vi "FT10_Fornax Switch Status Command.vi"(7 "Generator":T5="{\"Partition\":\"", 8 "Switch State":T1, 9 "Energy Channel ID":T2, 10 "Switch ID":T3, 11 "Source ID":T4) -> (3 "JSON Command":string)   [LabVIEW 2015]
uses:
  Controls/Control_Fornax Generator.ctl
  Controls/Control_Fornax Source ID.ctl
  Controls/Control_Fornax Switch ID.ctl
  Controls/Control_Fornax Energy Channel ID.ctl
  Controls/Control_Fornax Switch State.ctl
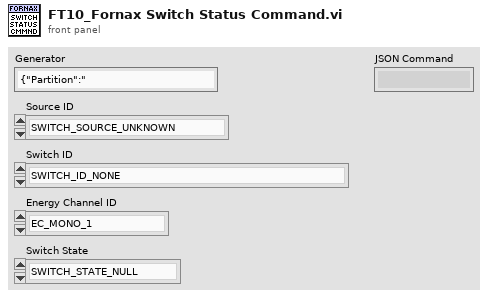
[diagram p1: front panel]
types:
  T1 = typedef "Control_Fornax Switch State.ctl" = enum16{"SWITCH_STATE_NULL  ", "SWITCH_STATE_PRESSED  ", "SWITCH_STATE_RELEASED  ", "NUM_SWITCH_STATES  "}
  T2 = typedef "Control_Fornax Energy Channel ID.ctl" = enum16{"EC_MONO_1  ", "EC_BIPOLAR  ", "EC_MONO_2  ", "EC_ADVANCED  ", "EC_ADVANCED_ECUT  ", "EC_ADVANCED_DCUT  ", "EC_SHARED_COAG  ", "EC_INTERNAL_BIP_CAL  "}
  T3 = typedef "Control_Fornax Switch ID.ctl" = enum16{"SWITCH_ID_NONE  ", "SWITCH_ID_CUT  ", "SWITCH_ID_VMODE  ", "SWITCH_ID_COAG  ", "SWITCH_ID_LIGASURE  ", "SWITCH_ID_BIPOLAR  ", "SWITCH_ID_STAPLER_CLOSE  ", "SWITCH_ID_STAPLER_OPEN  ", "SWITCH_ID_CARDIOBLATE_BIPOLAR  ", "SWITCH_ID_CARDIOBLATE_BIPOLAR_TOUCHSCREEN  ", "SWITCH_ID_CARDIOBLATE_MONOPOLAR  ", "SWITCH_ID_CARDIOBLATE_MONOPOLAR_TOUCHSCREEN  ", "SWITCH_ID_ULTRASONIC_BTN1  ", "SWITCH_ID_ULTRASONIC_BTN2  ", "SWITCH_ID_MAX  "}
  T4 = typedef "Control_Fornax Source ID.ctl" = enum16{"SWITCH_SOURCE_UNKNOWN  ", "SWITCH_SOURCE_HANDSWITCH  ", "SWITCH_SOURCE_FOOTSWITCH  ", "SWITCH_SOURCE_AUTO_BIPOLAR  ", "SWITCH_SOURCE_CARDIOBLATE  ", "SWITCH_SOURCE_SCREEN  ", "NUM_SWITCH_SOURCES  "}
  T5 = typedef "Control_Fornax Generator.ctl" = string
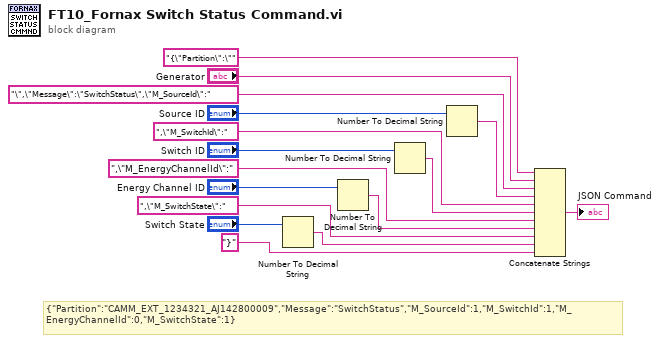
[diagram p0: block diagram]
diagram:
  # "{\"Partition\":\"CAMM_EXT_1234321_AJ142800009\",\"Message\":\"SwitchStatus\",\"M_SourceId\":1,\"M_SwitchId\":1,\"M_EnergyChannelId\":0,\"M_SwitchState\":1}"
  n1 = Number To Decimal String(number="Switch State") -> (decimal integer string=w14:string)  [unwired: 1 in]
  n2 = Number To Decimal String(number="Energy Channel ID") -> (decimal integer string=w11:string)  [unwired: 1 in]
  n3 = Number To Decimal String(number="Switch ID") -> (decimal integer string=w8:string)  [unwired: 1 in]
  n4 = Number To Decimal String(number="Source ID") -> (decimal integer string=w5:string)  [unwired: 1 in]
  n5 = Concatenate Strings("{\"Partition\":\"", "Generator", "\",\"Message\":\"SwitchStatus\",\"M_SourceId\":", w5, ",\"M_SwitchId\":", w8, ",\"M_EnergyChannelId\":", w11, ",\"M_SwitchState\":", w14, "}") -> (→"JSON Command":string)
